vi "Core Create.vi"(8 "error in (no error)":errorcluster, 10 "Plugin Name":string, 11 "CIFTemplateNode in":refnum<class "CIFTemplateNode.lvclass">) -> (0 "error out":errorcluster, 3 "CIFTemplateNode out":refnum<class "CIFTemplateNode.lvclass">)   [LabVIEW 2021, in "CIFTemplateNode.lvclass"]
uses:
  CIFTemplateNode.lvclass
  CIFTemplateCommon/Typedef/Plugin Status.ctl
  CIFTemplateCommon/Typedef/Plugin State.ctl
  CIFTemplateCommon/Typedef/Timing Statistics.ctl
  CIFTemplateCommon/Typedef/Timing Stats Base.ctl
  CIFTemplateCommon/Typedef/FIFO Statistics.ctl
  CIFTemplateCommon/Typedef/Simple Error.ctl
  CIFTemplateCommon/Typedef/Monitor Doubles.ctl
  CIFTemplateCommon/Typedef/Monitor U64.ctl
  CIFTemplateCommon/Typedef/Monitor I64.ctl
  CIFTemplateCommon/Typedef/Plugin Overrides.ctl
  CIFTemplateCommon/Typedef/Timing Overrides.ctl
  Typedef/Plugin Timestamps.ctl
  CIFUtilities/CIFOutOfBand/CIFOutOfBand.lvclass/CIFOutOfBand.ctl
  CIFTemplateNode.lvclass/CIFTemplateNode.ctl
  CIFTemplateCoreOOB/OOB_Rx/Private/Command Settings.vi
  CIFUtilities/CIFOutOfBand/Accessors/Write Local OOB Data.vi
  CIFTemplateCoreOOB/OOB_Tx/Private/Command Settings.vi
  CIFUtilities/CIFUtilities/Time/LabVIEW Time to UTC Time.vi
  CIFTemplateCoreOOB/OOB_Rx/CIFTemplateCoreOOB_Rx.lvclass
  D:/dev/CIF-LVCore/src/CIFUtilities/CIFOutOfBand/CIFOutOfBand.lvclass
  CIFTemplateCoreOOB/OOB_Tx/CIFTemplateCoreOOB_Tx.lvclass
  CIFUtilities/CIFOutOfBand/Init OOB.vi
  CIFTemplateCommon/CIFTemplateCommon.lvlib
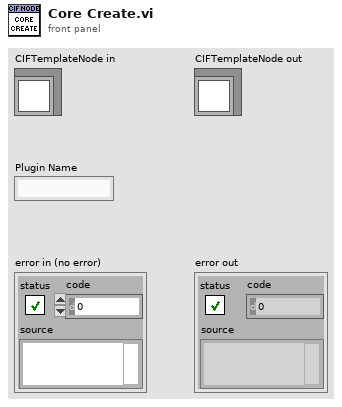
[diagram p1: front panel]
types:
  T1 = typedef "CIFTemplateNode.lvclass/Plugin Timestamps.ctl" = enum32{"Start Creation", "Start gRPC Servers", "Start Listening", "Start Running", "Wake", "Start Execute", "Read FIFO", "Write Output", "Cycle Execute", "Start Housekeeping", "Start Sleep", "Start Cleaningup", "Start Destroying"}
  T2 = typedef "CIFTemplateCommon.lvlib/Plugin Overrides.ctl" = cluster{"Timing Overrides":T3}
  T3 = typedef "CIFTemplateCommon.lvlib/Timing Overrides.ctl" = cluster{"Override Timing":bool, "Period (s)":dbl}
  T4 = typedef "CIFTemplateCommon.lvlib/Plugin Status.ctl" = cluster{"State":T5, "Timing Statistics (us)":T6, "FIFO Statistics (us)":T8, "error":T9, "Monitor Doubles":T10, "Monitor U64":T11, "Monitor I64":T12}
  T5 = typedef "CIFTemplateCommon.lvlib/Plugin State.ctl" = enum32{"Null", "Creating", "Listening", "Running", "CleaningUp", "Destroying"}
  T6 = typedef "CIFTemplateCommon.lvlib/Timing Statistics.ctl" = cluster{"Period":T7, "Wake Error":T7, "Execute":T7, "Housekeep":T7, "Idle":T7}
  T7 = typedef "CIFTemplateCommon.lvlib/Timing Stats Base.ctl" = cluster{"Max":i32, "Min":i32}
  T8 = typedef "CIFTemplateCommon.lvlib/FIFO Statistics.ctl" = cluster{"From T0":T7, "From Previous Plugin":T7, "Output Error":T7}
  T9 = typedef "CIFTemplateCommon.lvlib/Simple Error.ctl" = cluster{"status":bool, "code":i32}
  T10 = typedef "CIFTemplateCommon.lvlib/Monitor Doubles.ctl" = cluster{"1":dbl, "2":dbl, "3":dbl, "4":dbl}
  T11 = typedef "CIFTemplateCommon.lvlib/Monitor U64.ctl" = cluster{"1":u64, "2":u64, "3":u64, "4":u64}
  T12 = typedef "CIFTemplateCommon.lvlib/Monitor I64.ctl" = cluster{"1":i64, "2":i64, "3":i64, "4":i64}
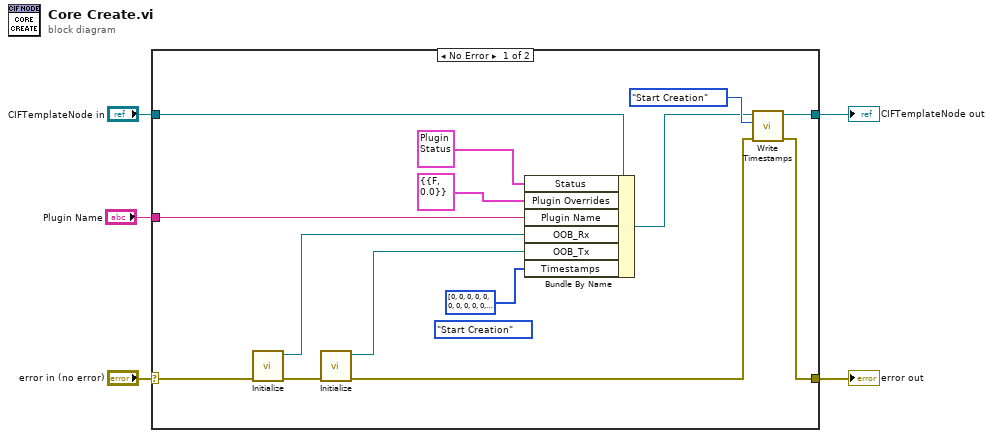
[diagram p0: block diagram]
diagram:
  n1 = case shown="No Error" "error in (no error)" {
    selector: "error in (no error)" -> [w12 w21]
    tunnel: [w9 w21] -> w4
    tunnel: [w7 w20] -> w2
    tunnel: "CIFTemplateNode in" -> [w11 w20]
    tunnel: "Plugin Name" -> [w6 _]
    frame No Error {
      (unwired) Plugin_Timestamps."Start Creation" ("Timestamps")
      n2 = call "Initialize.vi"("error in"=w12) -> ("error out"=w14:errorcluster, "CoreOOB_Rx out"=w16:refnum<class "CIFTemplateCoreOOB_Rx.lvclass">)  [unwired: 9 in]
      n3 = call "Initialize.vi"("error in"=w14) -> ("error out"=w10:errorcluster, "CoreOOB_Tx out"=w15:refnum<class "CIFTemplateCoreOOB_Tx.lvclass">)  [unwired: 9 in]
      n4 = Bundle By Name(cluster=w11, "Status"=T4 {"State"=enum."Creating", "Timing Statistics (us)"={"Period"={"Max"=0, "Min"=0}, "Wake Error"={"Max"=0, "Min"=0}, "Execute"={"Max"=0, "Min"=0}, "Housekeep"={"Max"=0, "Min"=0}, "Idle"={"Max"=0, "Min"=0}}, "FIFO Statistics (us)"={"From T0"={"Max"=0, "Min"=0}, "From Previous Plugin"={"Max"=0, "Min"=0}, "Output Error"={"Max"=0, "Min"=0}}, "error"={"status"=FALSE, "code"=0}, "Monitor Doubles"={"1"=0.0, "2"=0.0, "3"=0.0, "4"=0.0}, "Monitor U64"={"1"=0, "2"=0, "3"=0, "4"=0}, "Monitor I64"={"1"=0, "2"=0, "3"=0, "4"=0}}, "Plugin Overrides"=T2 {"Timing Overrides"={"Override Timing"=FALSE, "Period (s)"=0.0}}, "Plugin Name"=w6, "OOB_Rx"=w16, "OOB_Tx"=w15, "Timestamps"=u64[] [0, 0, 0, 0, 0, 0, 0, 0, 0, 0, 0, 0, 0]) -> (w8:refnum<class "CIFTemplateNode.lvclass">)
      n5 = call "Write Timestamps.vi"("error in (no error)"=w10, "Timestamp"=Plugin_Timestamps."Start Creation", "CIFTemplateNode in"=w8) -> ("error out"=w9:errorcluster, "CIFTemplateNode out"=w7:refnum<class "CIFTemplateNode.lvclass">)  [unwired: 7 in]
    }
    frame Error {
    }
  }
  "error out" <- w4
  "CIFTemplateNode out" <- w2
